vi "Configure Multiple Tone.vi"(0 "VISA resource name":refnum<visa-resource-name>, 1 "Enable Multiple Tones (T:Enable)":bool=TRUE, 5 "Initialize Phase (0: Fixed)":u16(ring) items=["Fixed", "Random"], 7 "Random Seed (0: Fixed)":u16(ring) items=["Fixed", "Random"], 9 "Frequency Spacing (10 kHz)":dbl=10000.0, 11 "error in (no error)":errorcluster, 12 "Number Of Tones (8)":i32=8, 13 "Alignment (1: Center)":u16(ring)=1 items=["Left", "Center", "Right"]) -> (4 "VISA resource name out":refnum<visa-resource-name>, 15 "error out":errorcluster)   [LabVIEW 2018, in "Agilent PSG MXG Series.lvlib"]
doc: "Initializes the phase for the multitone waveform, assigns the frequency spacing and defines the number of tones.\n\n<B>Notes:</B>\n(1) This VI is valid only in E8267C, E8267D, N5162A, N5182A, N5172B, N5182B.\n\n(2) For E8267C, this VI is valid only when the instrument installs <B>Option 002</B> (Internal baseband generator) or <B>Option 602</B> (Digital bus baseband generator).\n\n(3) For E8267D, this VI is valid only when the instrument installs <B>Option 601</B> or <B>Option 602</B> (Internal baseband generator).\n\n(4) For N5162A and N5182A, this VI is valid only when the instrument installs <B>Option 651</B> or <B>Option 652</B> or <B>Option 654</B> (Internal baseband generator), and <B>Option 430</B> (Multitone and two-tone)."
uses:
  Agilent PSG MXG Series.lvlib
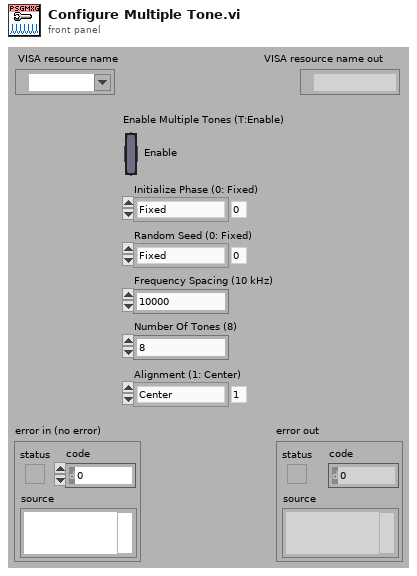
[diagram p1: front panel]
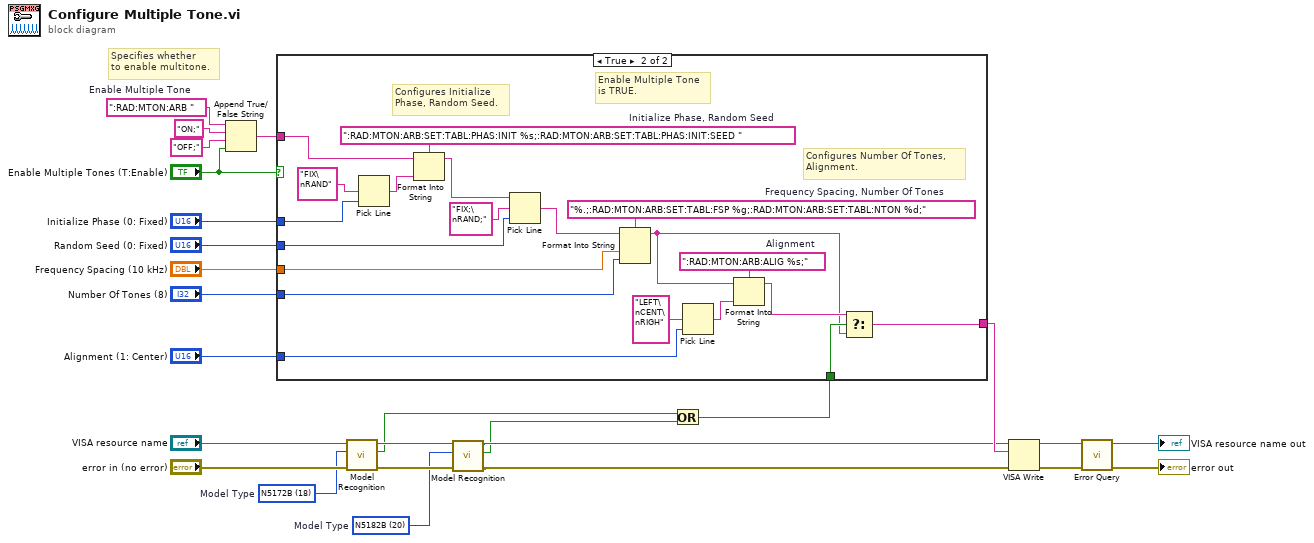
[diagram p0: block diagram]
diagram:
  w4 = u16 20 items=["N5181A"=0, "N5182A"=1, "N5183A"=2, "N5161A"=3, "N5162A"=4, "E8241A"=5, "E8244A"=6, "E8251A"=7, "E8254A"=8, "E8247C"=10, "E8257C"=11, "E8267C"=12, "E8257D"=15, "E8267D"=16, "N5171B"=17, "N5172B"=18, "N5181B"=19, "N5182B"=20, "N5173B"=21, "N5183B"=22]  # Model Type
  w5 = u16 18 items=["N5181A"=0, "N5182A"=1, "N5183A"=2, "N5161A"=3, "N5162A"=4, "E8241A"=5, "E8244A"=6, "E8251A"=7, "E8254A"=8, "E8247C"=10, "E8257C"=11, "E8267C"=12, "E8257D"=15, "E8267D"=16, "N5171B"=17, "N5172B"=18, "N5181B"=19, "N5182B"=20, "N5173B"=21, "N5183B"=22]  # Model Type
  w26 = ":RAD:MTON:ARB "  # Enable Multiple Tone
  # "Specifies whether\nto enable multitone."
  n1 = Append True/False String(1:"Enable Multiple Tones (T:Enable)", 2:"OFF;" ("false string"), 3:"ON;" ("true string"), 4:w26) -> (0:w23:string)
  n2 = call "Model Recognition.vi"("error in (no error)"="error in (no error)", "Model Type (0: N5181A)"=w5, "VISA resource name"="VISA resource name") -> ("error out"=w8:errorcluster, "Is Model Correct"=w3:bool, "VISA resource name out"=w9:refnum<visa-resource-name>)  [unwired: 6 in]
  n3 = call "Model Recognition.vi"("error in (no error)"=w8, "Model Type (0: N5181A)"=w4, "VISA resource name"=w9) -> ("error out"=w6:errorcluster, "Is Model Correct"=w2:bool, "VISA resource name out"=w7:refnum<visa-resource-name>)  [unwired: 6 in]
  n4 = Or(x=w3, y=w2) -> (x .or. y?=w1:bool)
  n5 = case shown="True" "Enable Multiple Tones (T:Enable)" {
    tunnel: w23 -> [w27 w47]
    tunnel: "Initialize Phase (0: Fixed)" -> [_ w43]
    tunnel: "Random Seed (0: Fixed)" -> [_ w40]
    tunnel: "Frequency Spacing (10 kHz)" -> [_ w37]
    tunnel: "Number Of Tones (8)" -> [_ w36]
    tunnel: "Alignment (1: Center)" -> [_ w32]
    tunnel: w1 -> [_ w31]
    tunnel: [w27 w30] -> w17
    frame False {
      # "Enable Multiple Tone\nis FALSE."
    }
    frame True {
      w35 = ":RAD:MTON:ARB:ALIG %s;"  # Alignment
      w38 = "%.;:RAD:MTON:ARB:SET:TABL:FSP %g;:RAD:MTON:ARB:SET:TABL:NTON %d;"  # Frequency Spacing, Number Of Tones
      w46 = ":RAD:MTON:ARB:SET:TABL:PHAS:INIT %s;:RAD:MTON:ARB:SET:TABL:PHAS:INIT:SEED "  # Initialize Phase, Random Seed
      # "Enable Multiple Tone\nis TRUE."
      # "Configures Number Of Tones,\nAlignment."
      # "Configures Initialize\nPhase, Random Seed."
      n6 = Pick Line(multi-line string="FIX\nRAND", line index=w43) -> (output string=w45:string)  [unwired: 1 out]
      n7 = Format Into String(format string=w46, initial string=w47, w45) -> (resulting string=w42:string)  [unwired: 1 in, 1 out]
      n8 = Pick Line(string ("")=w42, multi-line string="FIX;\nRAND;", line index=w40) -> (output string=w39:string)
      n9 = Format Into String(format string=w38, initial string=w39, w37, w36) -> (resulting string=w28:string)  [unwired: 1 in, 1 out]
      n10 = Pick Line(multi-line string="LEFT\nCENT\nRIGH", line index=w32) -> (output string=w34:string)  [unwired: 1 out]
      n11 = Format Into String(format string=w35, initial string=w28, w34) -> (resulting string=w29:string)  [unwired: 1 in, 1 out]
      n12 = Select(t=w29, s=w31, f=w28) -> (s? t:f=w30:string)
    }
  }
  n13 = VISA Write(VISA resource name=w7, write buffer=w17, error in (no error)=w6) -> (VISA resource name out=w16:refnum<visa-resource-name>, error out=w15:errorcluster)  [unwired: 1 out]
  n14 = call "Error Query.vi"("error in (no error)"=w15, "VISA resource name"=w16) -> ("error out"=→"error out":errorcluster, "VISA resource name out"=→"VISA resource name out":refnum<visa-resource-name>)  [unwired: 8 out]
